vi "EffectivePowerTest_RT.vi"() -> ()   [LabVIEW 2016]
uses:
  <vilib>/userdefined/High Color/nirio_resource_hc.ctl
  <vilib>/myRIO/Common/Instrument Driver Framework/myRIO v1.0/UART/vis/myRIO v1.0 Close UART.vi
  <vilib>/FPGAPlugInAG/myRIO-1900/niLvFpga_Open_myRIO-1900.vi
  <vilib>/rvi/interface/common/dynamic/niFpgaDynamicAddResources.vi
  <vilib>/Utility/file.llb/Read Delimited Spreadsheet (DBL).vi
  <vilib>/Utility/error.llb/Error Cluster From Error Code.vi
  <vilib>/rvi/errors/niLvFpgaAdjustHostInterfaceError.vi
  <vilib>/FPGAPlugInAG/Dynamic/niLvFpga_Close_Dynamic.vi
  <vilib>/myRIO/Common/Instrument Driver Framework/Utilities/vis/FPGA Ref Manager.vi
  <vilib>/myRIO/Common/Instrument Driver Framework/myRIO v1.0/myRIO v1.0 Reset FPGA.vi
  <vilib>/myRIO/Common/Instrument Driver Framework/myRIO v1.0/IRQ/vis/myRIO v1.0 IRQ Info FGV.vi
  <vilib>/myRIO/Common/Instrument Driver Framework/myRIO v1.0/IRQ/vis/myRIO v1.0 Timer IRQ Info FGV.vi
  <vilib>/myRIO/Common/Instrument Driver Framework/myRIO v1.0/IRQ/vis/myRIO v1.0 ISR Agent.vi
  <vilib>/rvi/interface/nirviOpenFPGA/nirviOpenFPGA.xnode
  FPGA Bitfiles/Dymin4ALL_FPGATarget_EffectivePowerTe_1xxxSxpVT6U.lvbitx
  EffectivePowerTest.vi
  <vilib>/rvi/interface/nirviReadWriteControl/nirviReadWriteControl.xnode
  <vilib>/rvi/interface/nirviCloseFPGA/nirviCloseFPGA.xnode
  NiFpgaLv.dll
  <vilib>/rvi/interface/Simulation/niFpgaSimulationCallBeginRW.vi
  <vilib>/myRIO/Instrument Drivers/Utilities/Utilities.lvlib
panel:
  out "Step Times (bits)":i32[](array[numeric])
  out "AOM bits":u16[](array[numeric])
  in  "stop":bool
  out "Fit Parameters":dbl[](array[numeric])
  out "error out":errorcluster
  out "All Step Times (bits)":i32[](array[numeric])
  in  "Laser Wait time (us)":dbl
  in  "DyMIN Step Times (us)":dbl[](array[numeric])=[0.0, 0.0, 0.0, 0.0] min=0.0 max=10000.0 step=0.0125
  out "AOM Voltage":dbl[](array[numeric])
  in  "DyMIN Step Power (mW)":dbl[](array[numeric])=[0.0, 0.0, 0.0, 0.0] min=0.0 max=1.0
  in  "YYMMDD of last calibration":string
  in  "OK":bool
  out "Input needed":bool
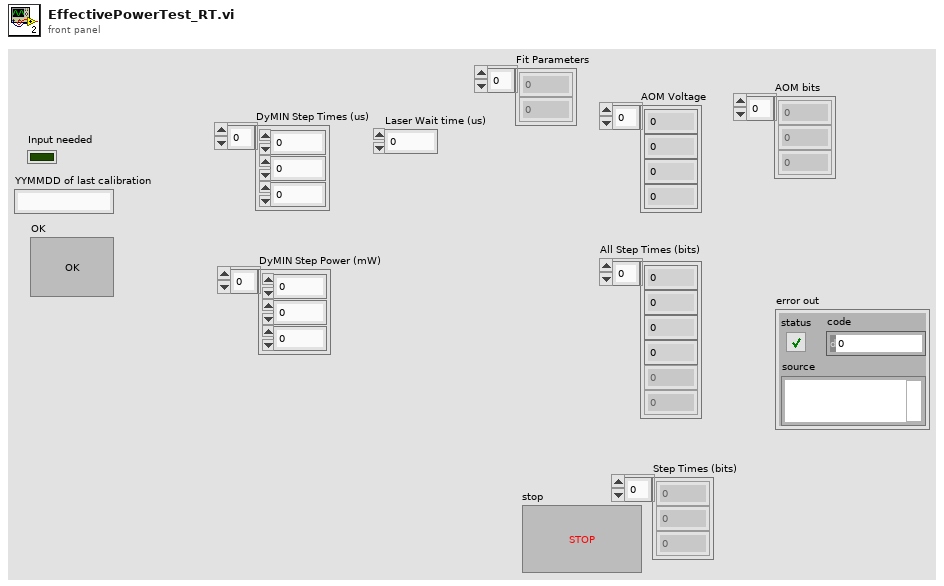
[diagram p1: front panel]
types:
  T1 = typedef "nirio_resource_hc.ctl" = tag
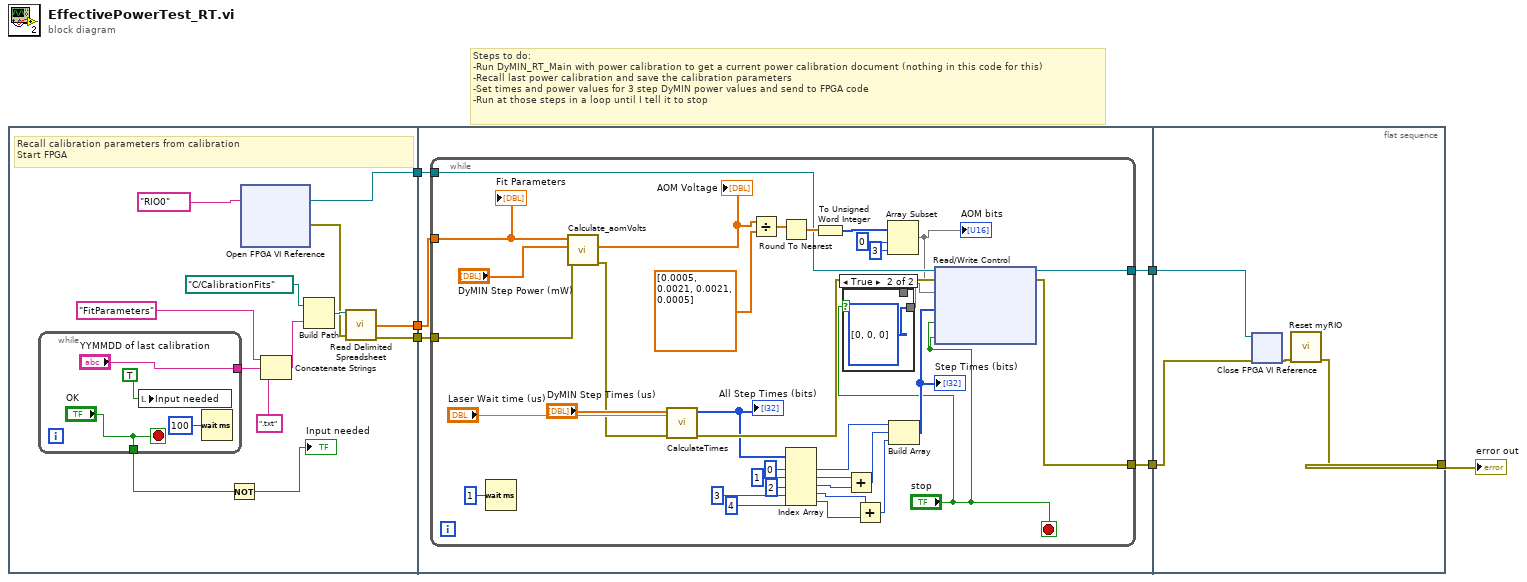
[diagram p0: block diagram]
diagram:
  # "Steps to do:\n-Run DyMIN_RT_Main with power calibration to get a current power calibration document (nothing in this code for this)\n-Recall last power calibration and save the calibration parameters\n-Set times and power values for 3 step DyMIN power values and send to FPGA code\n-Run at those steps in a loop until I tell it to stop"
  n1 = flat-sequence {
    tunnel: [w11] -> w6
    tunnel: [w10] -> w5
    tunnel: [w7] -> w4
    tunnel: w6 -> [w28]
    tunnel: w5 -> [w27]
    tunnel: w4 -> [w26]
    tunnel: [w25] -> w2
    tunnel: [w24] -> w1
    tunnel: [w66] -> w3
    tunnel: w2 -> [w67]
    tunnel: w1 -> [w68]
    frame #0 {
      # "Recall calibration parameters from calibration\nStart FPGA"
      n2 = while {
        tunnel: ["YYMMDD of last calibration"] -> w14
        tunnel: ["OK"] -> w13
        stop <- "OK" stop-if-true
        n3 = local write "Input needed"(TRUE ("Input needed")) -> ()
        n4 = Wait (ms)(milliseconds to wait=u32 100) -> ()  [unwired: 1 out]
      }
      n5 = Not(x=w13) -> (.not. x?=→"Input needed":bool)
      n6 = xnode "Open FPGA VI Reference"("resource name"=T1 "RIO0") -> ("FPGA VI Reference Out"=w7:refnum<k20>, "error out"=w8:errorcluster)  [unwired: 1 in]
      n7 = Concatenate Strings("FitParameters", w14, ".txt" ("string")) -> (w16:string)
      n8 = Build Path(base path=path "C:/CalibrationFits", name or relative path=w16) -> (appended path=w15:path)
      n9 = call-poly <vilib>:"Read Delimited Spreadsheet.vi"("file path (dialog if empty)"=w15, "error in (no error)"=w8) -> ("first row"=w11:dbl[], "error out"=w10:errorcluster)  [unwired: 8 in, 4 out]
    }
    frame #1 {
      n10 = while {
        tunnel: w28 -> [w63]
        tunnel: w27 -> [w62]
        tunnel: w26 -> [w52]
        tunnel: [w50] -> w25
        tunnel: [w29] -> w24
        stop <- "stop" stop-if-true
        n11 = Wait (ms)(milliseconds to wait=u32 1) -> ()  [unwired: 1 out]
        n12 = call "Calculate_aomVolts.vi"("error in (no error)"=w62, "Power"="DyMIN Step Power (mW)", "Fit Parameters"=w63) -> ("error out"=w54:errorcluster, "AOM Voltage"=w60:dbl[])  [unwired: 7 in]
        "AOM Voltage" <- w60
        n13 = call "CalculateTimes.vi"("error in"=w54, "Laser Wait time (us)"="Laser Wait time (us)", "DyMIN Step Times (us)"="DyMIN Step Times (us)") -> ("error out"=w51:errorcluster, "All Step Times (bits)"=w46:i32[])  [unwired: 3 in, 4 out]
        "All Step Times (bits)" <- w46
        n14 = Divide(x=w60, y=dbl[] [0.0005, 0.0021, 0.0021, 0.0005]) -> (x/y=w58:dbl[])
        n15 = Round To Nearest(number=w58) -> (nearest integer value=w57:dbl[])
        n16 = Index Array(array=w46, index #1=0 ("index"), index #2=1 ("index"), index #3=2 ("index"), index #4=3 ("index"), index #5=4 ("index")) -> (element #1=w37:i32, element #2=w35:i32, element #3=w36:i32, element #4=w33:i32, element #5=w34:i32)
        n17 = To Unsigned Word Integer(number=w57) -> (unsigned 16bit integer=w49:u16[])
        n18 = Add(x=w35, y=w36) -> (x+y=w41:i32)
        n19 = Add(x=w33, y=w34) -> (x+y=w40:i32)
        n20 = Array Subset(array=w49, index=0, length=3) -> (w32:u16[])
        "AOM bits" <- w32
        n21 = case shown="True" "stop" {
          tunnel: w32 -> [w64 _]
          tunnel: [w64 u16[] [0, 0, 0]] -> w31
          frame False {
          }
          frame True {
          }
        }
        n22 = Build Array(w37, w41, w40) -> (w38:i32[])
        "Step Times (bits)" <- w38
        n23 = xnode "Read/Write Control"("FPGA VI Reference In"=w52, "error in"=w51, "AOM Volt (bits)"=w31, "Step Times (bits"=w38, "End Program"="stop", "End Program 2"="stop") -> ("FPGA VI Reference Out"=w29:refnum<k20>, "error out"=w50:errorcluster)
        "Fit Parameters" <- w63
      }
    }
    frame #2 {
      n24 = xnode "Close FPGA VI Reference"("FPGA VI Reference In"=w68, "error in"=w67) -> ("error out"=w69:errorcluster)
      n25 = call <vilib>:"Reset myRIO.vi"("error in (no error)"=w69) -> ("error out"=w66:errorcluster)  [unwired: 10 in]
    }
  }
  "error out" <- w3
